vi "mqttCmdConnectStatusRead.vi"(0 "mqttConnect in":refnum<class "mqttCmdConnect.lvclass">, 11 "error in (no error)":errorcluster) -> (4 "mqttConnect out":refnum<class "mqttCmdConnect.lvclass">, 6 "connStatus":T1=enum."Connection refused: not authorized", 15 "error out":errorcluster)   [LabVIEW 2013, in "mqttCmdConnect.lvclass"]
uses:
  mqttCmdConnect.lvclass
  mqttTypedef/mqttConnectionStatus.ctl
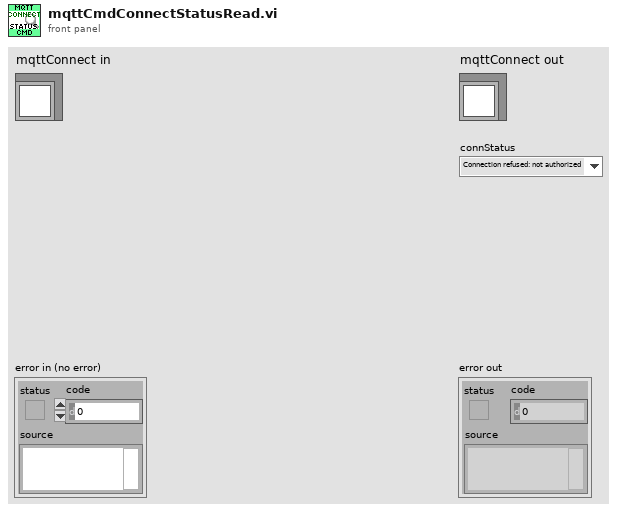
[diagram p1: front panel]
types:
  T1 = typedef "mqttConnectionStatus.ctl" = enum16{"Connection accepted", "Connection refused: unacceptable protocol version", "Connection refused: identifier rejected", "Connection refused: Server unavailable", "Connection refused: bad user name or password", "Connection refused: not authorized"}
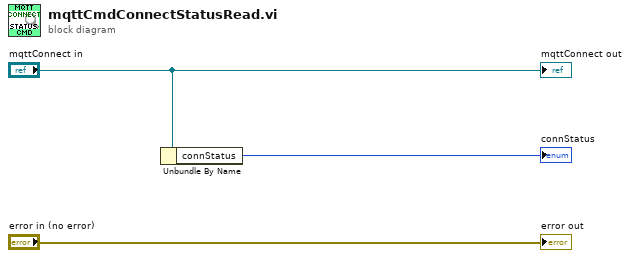
[diagram p0: block diagram]
diagram:
  n1 = Unbundle By Name("mqttConnect in") -> ("connStatus"=→"connStatus":T1)
  "error out" <- "error in (no error)"
  "mqttConnect out" <- "mqttConnect in"
